vi "Create FP Item.vi"(6 "Cluster Component":bool, 8 "error in (no error)":errorcluster, 10 "GObject In":refnum<vi>, 11 "GText in":refnum<class "Text.lvclass">) -> (0 "error out":errorcluster, 1 "Is Control":bool, 2 "Is Indicator":bool, 3 "GText out":refnum<class "Text.lvclass">, 4 "All Objects Created":refnum<class "Object.lvclass">[](array[class]), 5 "Is Visible":bool)   [LabVIEW 2017, in "Front Panel Publisher.lvlib" / "Text.lvclass"]
uses:
  Text.lvclass
  Enum - Create Text Method.ctl
  Object_class/Object.lvclass
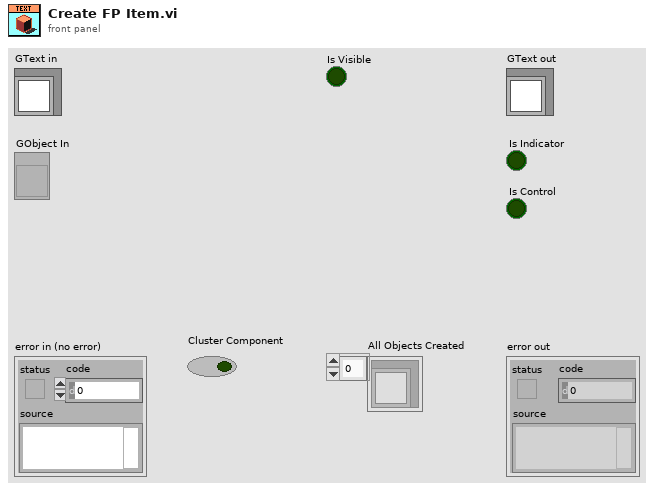
[diagram p1: front panel]
types:
  T1 = typedef "Front Panel Publisher.lvlib/Text.lvclass/Enum - Create Text Method.ctl" = enum16{"Text", "Label", "Caption", "Boolean Text"}
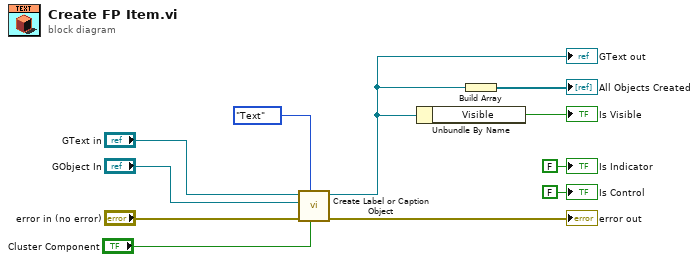
[diagram p0: block diagram]
diagram:
  n1 = call "Create Label or Caption Object.vi"("Cluster Component"="Cluster Component", "Text Type"=Enum_-_Create_Text_Method."Text", "error in (no error)"="error in (no error)", "GObject"="GObject In", "Text in"="GText in") -> ("error out"=→"error out":errorcluster, "Text out"=w3:refnum<class "Text.lvclass">)  [unwired: 5 in]
  "GText out" <- w3
  n2 = Unbundle By Name(w3) -> ("Visible"=→"Is Visible":bool)
  n3 = Build Array(w3) -> (→"All Objects Created":refnum<class "Text.lvclass">[])
  "Is Indicator" <- FALSE ("Is Indicator")
  "Is Control" <- FALSE ("Is Control")
